vi "InstrumentSelection.vi"(8 "error in (no error)":errorcluster, 9 "Verify GPIB address":bool, 10 "Instrument type":T1(ring), 11 "Instrument name IN":string(combo)) -> (0 "error out":errorcluster, 1 "Instrument name OUT":string, 2 "LCR":refnum<class "LCRControl.lvclass">, 3 "Supply":refnum<class "SupplyControl.lvclass">, 4 "Switching":refnum<class "Switching.lvclass">, 5 "Multimeter":refnum<class "MultimeterControl.lvclass">)   [LabVIEW 2019, in "InstrControl.lvclass"]
uses:
  InstrControl.lvclass
  SupplyControl/SupplyControl.lvclass
  C:/Users/Semiprobe/Desktop/Probe-Test-Software/itk-strip-sensor-qc/LabVIEW 2019/InstrControl/InstrControl.lvclass
  LCRControl/LCRControl.lvclass
  MultimeterControl/MultimeterControl.lvclass
  Switching/Switching.lvclass
  SupplyControl/Keithley 2410/KE2410.lvclass
  C:/Users/Semiprobe/Desktop/Probe-Test-Software/itk-strip-sensor-qc/LabVIEW 2019/InstrControl/SupplyControl/SupplyControl.lvclass
  SupplyControl/Keithley 2657A/KE2657A.lvclass
  SupplyControl/Keithley 6517/KE6517.lvclass
  SupplyControl/Keithley 487/KE487.lvclass
  SupplyControl/Keithley 236 & 237/KE236.lvclass
  LCRControl/WK6440B/WK6440B.lvclass
  C:/Users/Semiprobe/Desktop/Probe-Test-Software/itk-strip-sensor-qc/LabVIEW 2019/InstrControl/LCRControl/LCRControl.lvclass
  LCRControl/WK6425/WK6425.lvclass
  MultimeterControl/Keithley 2000/KE2000.lvclass
  C:/Users/Semiprobe/Desktop/Probe-Test-Software/itk-strip-sensor-qc/LabVIEW 2019/InstrControl/MultimeterControl/MultimeterControl.lvclass
  Switching/Pickering/Pickering.lvclass
  C:/Users/Semiprobe/Desktop/Probe-Test-Software/itk-strip-sensor-qc/LabVIEW 2019/InstrControl/Switching/Switching.lvclass
  Switching/Keithley 3706A/KE3706A.lvclass
  Switching/LXIPXISwitching/LXIPXISwitching.lvclass
  InstrumentSetup.vi
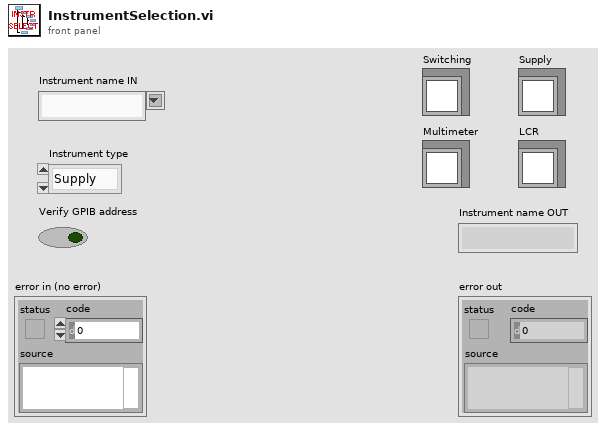
[diagram p1: front panel]
types:
  T1 = enum16{"Supply", "LCR", "Multimeter", "Switching"}
  T2 = cluster{"KE 2410":cluster{"Instrument name":string, "address":refnum<visa-resource-name>, "Instrument type":u16}, "KE 6517":cluster{"Instrument name":string, "address":refnum<visa-resource-name>, "Instrument type":u16}, "KE 487":cluster{"Instrument name":string, "address":refnum<visa-resource-name>, "Instrument type":u16}, "KE 236":cluster{"Instrument name":string, "address":refnum<visa-resource-name>, "Instrument type":u16}, "WK 6440B":cluster{"Instrument name":string, "address":refnum<visa-resource-name>, "Instrument type":u16}, "WK 6425":cluster{"Instrument name":string, "address":refnum<visa-resource-name>, "Instrument type":u16}, "Pickering Matrix":cluster{"Instrument name":string, "address":refnum<visa-resource-name>, "Instrument type":u16}, "KE 2000":cluster{"Instrument name":string, "address":refnum<visa-resource-name>, "Instrument type":u16}, "KE3706A Switching":cluster{"Instrument name":string, "address":refnum<visa-resource-name>, "Instrument type":u16}, "KE 2657A":cluster{"Instrument name":string, "address":refnum<visa-resource-name>, "Instrument type":u16}}
  T3 = cluster{"Current Limit":sgl, "KE2410":refnum<class "KE2410.lvclass">}
  T4 = cluster{"Current Limit":sgl, "KE2657A":refnum<class "KE2657A.lvclass">}
  T5 = cluster{"Current Limit":u16, "KE6517":refnum<class "KE6517.lvclass">}
  T6 = cluster{"Compliance":u16, "Range:":u16, "KE487":refnum<class "KE487.lvclass">}
  T7 = cluster{"current \ncompliance level":dbl, "compliance/\nmeasurement range (auto:0)":u16, "KE236":refnum<class "KE236.lvclass">}
  T8 = cluster{"RC Configuration":u16, "AC amplitude [V]":dbl, "AC frequency [Hz]":i32, "WK6440B":refnum<class "WK6440B.lvclass">}
  T9 = cluster{"RC Configuration":u16, "AC amplitude [V]":dbl, "AC frequency [Hz]":i32, "WK6425":refnum<class "WK6425.lvclass">}
  T10 = cluster{"Range":u16, "Range Value":dbl, "Function":u16, "KE2000":refnum<class "KE2000.lvclass">}
  T11 = cluster{"Matrix address":string, "Mux1 address":string, "Mux2 address":string, "Pickering":refnum<class "Pickering.lvclass">, "Matrix X Channels":cluster{"Bias Supply / SMU LO":i32, "Bias Supply / SMU HI":i32, "CV Box LO":i32, "CV Box HI":i32, "CV Box LO IN":i32, "CV Box HI IN":i32, "Volt meter LO":i32, "Volt meter HI":i32, "Mux1 C1":i32, "Mux1 C2":i32, "Mux2 C1":i32, "Mux2 C2":i32}}
  T12 = cluster{"Mux1 slot":string, "Mux2 slot":string, "KE3706A":refnum<class "KE3706A.lvclass">}
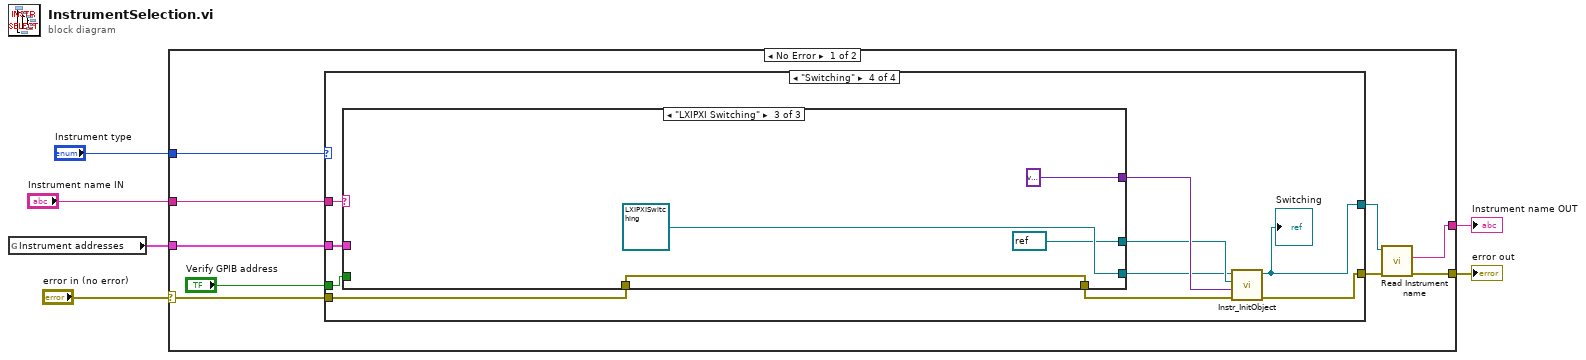
[diagram p0: block diagram]
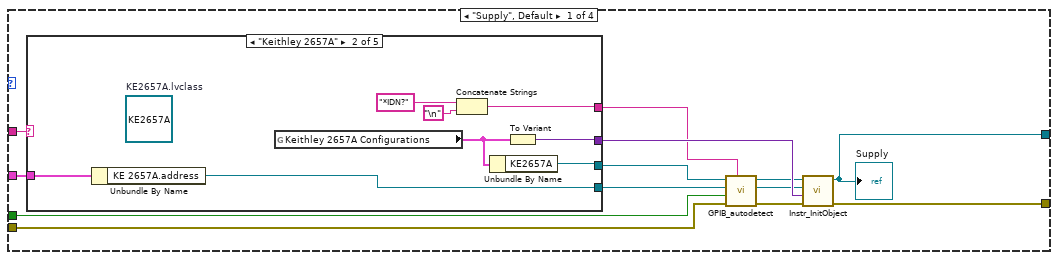
[diagram p2: hidden frame]
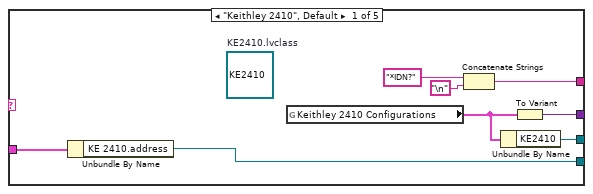
[diagram p3: hidden frame]
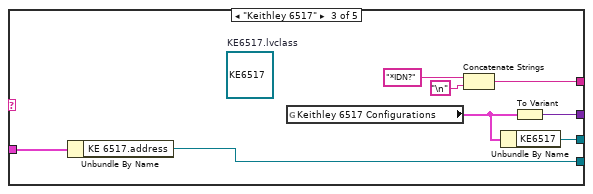
[diagram p4: hidden frame]
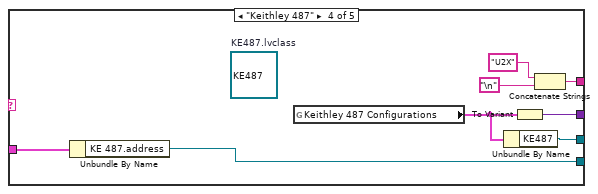
[diagram p5: hidden frame]
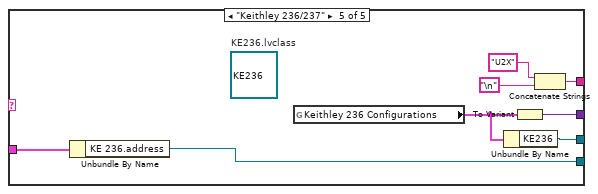
[diagram p6: hidden frame]
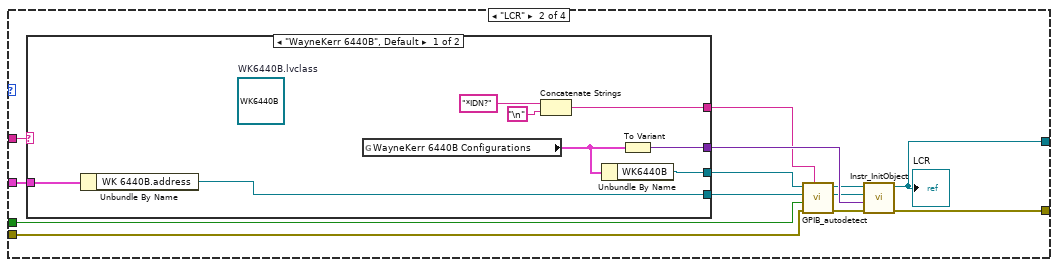
[diagram p7: hidden frame]
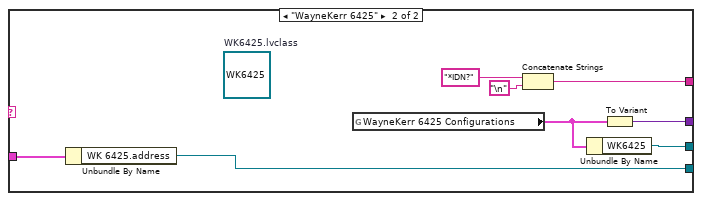
[diagram p8: hidden frame]
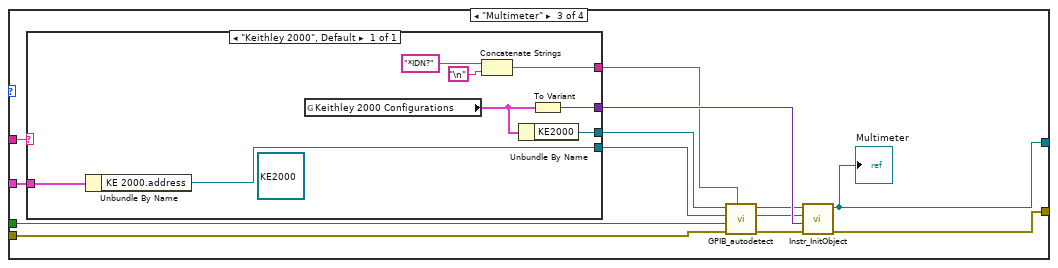
[diagram p9: hidden frame]
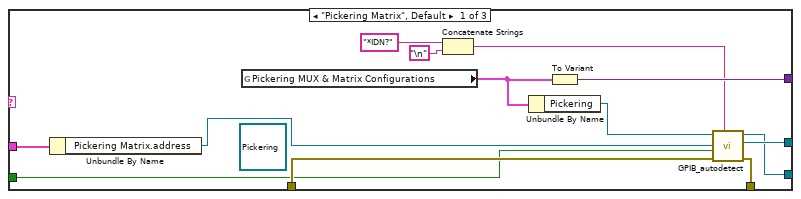
[diagram p10: hidden frame]
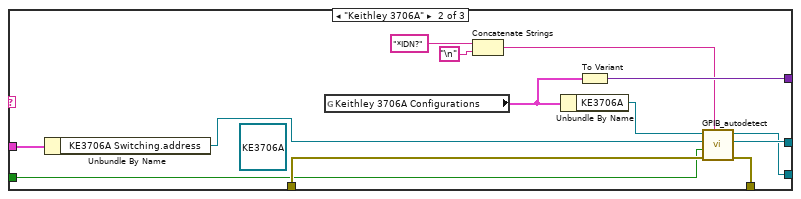
[diagram p11: hidden frame]
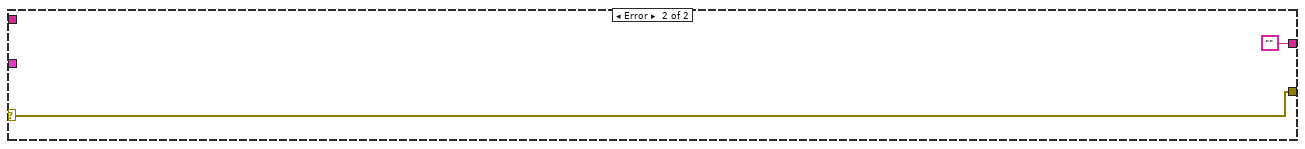
[diagram p12: hidden frame]
diagram:
  n1 = global read "InstrumentSetup.vi" "Instrument addresses"() -> (w1:T2)
  n2 = case shown="No Error" "error in (no error)" {
    selector: "error in (no error)" -> [w13 w160]
    tunnel: [w14 w160] -> w5
    tunnel: [w15 ""] -> w4
    tunnel: "Instrument type" -> [w10 _]
    tunnel: "Instrument name IN" -> [w9 _]
    tunnel: w1 -> [w8 _]
    frame No Error {
      n3 = case shown="\"Switching\"" w10 {
        tunnel: w9 -> [w28 w81 w110 w125]
        tunnel: [w27 w79 w108 w127] -> w12
        tunnel: w13 -> [w19 w76 w100 w123]
        tunnel: [w26 w80 w109 w128] -> w11
        tunnel: w8 -> [w25 w78 w107 w126]
        tunnel: "Verify GPIB address" -> [w18 w70 w105 w122]
        frame "Supply", Default {
          n4 = case shown="\"Keithley 2657A\"" w28 {
            tunnel: [w33 w39 w48 w56 w64] -> w21
            tunnel: w25 -> [w36 w38 w52 w60 w68]
            tunnel: [w35 w37 w51 w59 w67] -> w23
            tunnel: [w34 w40 w50 w58 w66] -> w24
            tunnel: [w29 w41 w45 w53 w61] -> w16
            frame "Keithley 2410", Default {
              (unwired) refnum<class "KE2410.lvclass"> refnum  # KE2410.lvclass
              n5 = Unbundle By Name(w36) -> ("KE 2410.address"=w35:refnum<visa-resource-name>)
              n6 = global read "InstrumentSetup.vi" "Keithley 2410 Configurations"() -> (w32:T3)
              n7 = Concatenate Strings("*IDN?" ("regular expression"), "\n") -> (w29:string)
              n8 = Unbundle By Name(w32) -> ("KE2410"=w33:refnum<class "KE2410.lvclass">)
              n9 = To Variant(anything=w32) -> (Variant=w34:variant)
            }
            frame "Keithley 2657A" {
              (unwired) refnum<class "KE2657A.lvclass"> refnum  # KE2657A.lvclass
              n10 = Unbundle By Name(w38) -> ("KE 2657A.address"=w37:refnum<visa-resource-name>)
              n11 = global read "InstrumentSetup.vi" "Keithley 2657A Configurations"() -> (w44:T4)
              n12 = Concatenate Strings("*IDN?" ("regular expression"), "\n") -> (w41:string)
              n13 = Unbundle By Name(w44) -> ("KE2657A"=w39:refnum<class "KE2657A.lvclass">)
              n14 = To Variant(anything=w44) -> (Variant=w40:variant)
            }
            frame "Keithley 6517" {
              (unwired) refnum<class "KE6517.lvclass"> refnum  # KE6517.lvclass
              n15 = Unbundle By Name(w52) -> ("KE 6517.address"=w51:refnum<visa-resource-name>)
              n16 = global read "InstrumentSetup.vi" "Keithley 6517 Configurations"() -> (w49:T5)
              n17 = Concatenate Strings("*IDN?" ("regular expression"), "\n") -> (w45:string)
              n18 = Unbundle By Name(w49) -> ("KE6517"=w48:refnum<class "KE6517.lvclass">)
              n19 = To Variant(anything=w49) -> (Variant=w50:variant)
            }
            frame "Keithley 487" {
              (unwired) refnum<class "KE487.lvclass"> refnum  # KE487.lvclass
              n20 = Unbundle By Name(w60) -> ("KE 487.address"=w59:refnum<visa-resource-name>)
              n21 = global read "InstrumentSetup.vi" "Keithley 487 Configurations"() -> (w57:T6)
              n22 = Unbundle By Name(w57) -> ("KE487"=w56:refnum<class "KE487.lvclass">)
              n23 = To Variant(anything=w57) -> (Variant=w58:variant)
              n24 = Concatenate Strings("U2X" ("regular expression"), "\n") -> (w53:string)
            }
            frame "Keithley 236/237" {
              (unwired) refnum<class "KE236.lvclass"> refnum  # KE236.lvclass
              n25 = Unbundle By Name(w68) -> ("KE 236.address"=w67:refnum<visa-resource-name>)
              n26 = global read "InstrumentSetup.vi" "Keithley 236 Configurations"() -> (w65:T7)
              n27 = Unbundle By Name(w65) -> ("KE236"=w64:refnum<class "KE236.lvclass">)
              n28 = To Variant(anything=w65) -> (Variant=w66:variant)
              n29 = Concatenate Strings("U2X" ("regular expression"), "\n") -> (w61:string)
            }
          }
          n30 = call-dynamic "GPIB_autodetect.vi"("ID command"=w16, "error in (no error)"=w19, "Verify GPIB address"=w18, "Instrument address in"=w23, "InstrControl in"=w21) -> ("error out"=w17:errorcluster, "Instrument address out"=w22:refnum<visa-resource-name>, "InstrControl out"=w20:refnum<class "SupplyControl.lvclass">)  [unwired: 4 in]
          n31 = call-dynamic "Instr_InitObject.vi"("error in (no error)"=w17, "Instrument Configuration"=w24, "Instrument address"=w22, "SupplyControl in"=w20) -> ("error out"=w26:errorcluster, "SupplyControl out"=w27:refnum<class "SupplyControl.lvclass">)  [unwired: 6 in]
          "Supply" <- w27
        }
        frame "LCR" {
          n32 = case shown="\"WayneKerr 6440B\", Default" w81 {
            tunnel: [w85 w93] -> w72
            tunnel: w78 -> [w89 w97]
            tunnel: [w88 w96] -> w74
            tunnel: [w87 w95] -> w77
            tunnel: [w82 w90] -> w69
            frame "WayneKerr 6440B", Default {
              (unwired) refnum<class "WK6440B.lvclass"> refnum  # WK6440B.lvclass
              n33 = Unbundle By Name(w89) -> ("WK 6440B.address"=w88:refnum<visa-resource-name>)
              n34 = global read "InstrumentSetup.vi" "WayneKerr 6440B Configurations"() -> (w86:T8)
              n35 = Concatenate Strings("*IDN?" ("regular expression"), "\n") -> (w82:string)
              n36 = Unbundle By Name(w86) -> ("WK6440B"=w85:refnum<class "WK6440B.lvclass">)
              n37 = To Variant(anything=w86) -> (Variant=w87:variant)
            }
            frame "WayneKerr 6425" {
              (unwired) refnum<class "WK6425.lvclass"> refnum  # WK6425.lvclass
              n38 = Unbundle By Name(w97) -> ("WK 6425.address"=w96:refnum<visa-resource-name>)
              n39 = global read "InstrumentSetup.vi" "WayneKerr 6425 Configurations"() -> (w94:T9)
              n40 = Concatenate Strings("*IDN?" ("regular expression"), "\n") -> (w90:string)
              n41 = Unbundle By Name(w94) -> ("WK6425"=w93:refnum<class "WK6425.lvclass">)
              n42 = To Variant(anything=w94) -> (Variant=w95:variant)
            }
          }
          n43 = call-dynamic "GPIB_autodetect.vi"("ID command"=w69, "error in (no error)"=w76, "Verify GPIB address"=w70, "Instrument address in"=w74, "InstrControl in"=w72) -> ("error out"=w75:errorcluster, "Instrument address out"=w73:refnum<visa-resource-name>, "InstrControl out"=w71:refnum<class "LCRControl.lvclass">)  [unwired: 4 in]
          n44 = call-dynamic "Instr_InitObject.vi"("error in (no error)"=w75, "Instrument Configuration"=w77, "Instrument address"=w73, "LCRControl in"=w71) -> ("error out"=w80:errorcluster, "LCRControl out"=w79:refnum<class "LCRControl.lvclass">)  [unwired: 6 in]
          "LCR" <- w79
        }
        frame "Multimeter" {
          n45 = case shown="\"Keithley 2000\", Default" w110 {
            tunnel: [w114] -> w101
            tunnel: w107 -> [w118]
            tunnel: [w117] -> w104
            tunnel: [w116] -> w106
            tunnel: [w111] -> w98
            frame "Keithley 2000", Default {
              (unwired) refnum<class "KE2000.lvclass"> refnum ("KE2000.lvclass")
              n46 = Unbundle By Name(w118) -> ("KE 2000.address"=w117:refnum<visa-resource-name>)
              n47 = global read "InstrumentSetup.vi" "Keithley 2000 Configurations"() -> (w115:T10)
              n48 = Concatenate Strings("*IDN?" ("regular expression"), "\n") -> (w111:string)
              n49 = Unbundle By Name(w115) -> ("KE2000"=w114:refnum<class "KE2000.lvclass">)
              n50 = To Variant(anything=w115) -> (Variant=w116:variant)
            }
          }
          n51 = call-dynamic "GPIB_autodetect.vi"("ID command"=w98, "error in (no error)"=w100, "Verify GPIB address"=w105, "Instrument address in"=w104, "InstrControl in"=w101) -> ("error out"=w99:errorcluster, "Instrument address out"=w103:refnum<visa-resource-name>, "InstrControl out"=w102:refnum<class "KE2000.lvclass">)  [unwired: 4 in]
          n52 = call-dynamic "Instr_InitObject.vi"("error in (no error)"=w99, "Instrument Configuration"=w106, "Instrument address"=w103, "KE2000 in"=w102) -> ("error out"=w109:errorcluster, "KE2000 out"=w108:refnum<class "KE2000.lvclass">)  [unwired: 6 in]
          "Multimeter" <- w108
        }
        frame "Switching" {
          n53 = case shown="\"LXIPXI Switching\"" w125 {
            tunnel: w126 -> [w141 w152 _]
            tunnel: [w139 w151 variant ("Variant")] -> w124
            tunnel: w123 -> [w135 w149 w155]
            tunnel: w122 -> [w134 w142 _]
            tunnel: [w131 w148 w155] -> w121
            tunnel: [w130 w145 refnum<visa-resource-name> refnum ("Instrument address out")] -> w120
            tunnel: [w129 w144 refnum<class "LXIPXISwitching.lvclass"> refnum ("LXIPXISwitching.lvclass")] -> w119
            frame "Pickering Matrix", Default {
              (unwired) refnum<class "Pickering.lvclass"> refnum ("Pickering")
              n54 = Unbundle By Name(w141) -> ("Pickering Matrix.address"=w133:refnum<visa-resource-name>)
              n55 = global read "InstrumentSetup.vi" "Pickering MUX & Matrix Configurations"() -> (w140:T11)
              n56 = Concatenate Strings("*IDN?" ("regular expression"), "\n") -> (w136:string)
              n57 = Unbundle By Name(w140) -> ("Pickering"=w132:refnum<class "Pickering.lvclass">)
              n58 = To Variant(anything=w140) -> (Variant=w139:variant)
              n59 = call-dynamic "GPIB_autodetect.vi"("ID command"=w136, "error in (no error)"=w135, "Verify GPIB address"=w134, "Instrument address in"=w133, "InstrControl in"=w132) -> ("error out"=w131:errorcluster, "Instrument address out"=w130:refnum<visa-resource-name>, "InstrControl out"=w129:refnum<class "Pickering.lvclass">)  [unwired: 4 in]
            }
            frame "Keithley 3706A" {
              (unwired) refnum<class "KE3706A.lvclass"> refnum ("KE3700A in")
              n60 = Unbundle By Name(w152) -> ("KE3706A Switching.address"=w146:refnum<visa-resource-name>)
              n61 = global read "InstrumentSetup.vi" "Keithley 3706A Configurations"() -> (w154:T12)
              n62 = Concatenate Strings("*IDN?" ("regular expression"), "\n") -> (w143:string)
              n63 = Unbundle By Name(w154) -> ("KE3706A"=w147:refnum<class "KE3706A.lvclass">)
              n64 = To Variant(anything=w154) -> (Variant=w151:variant)
              n65 = call-dynamic "GPIB_autodetect.vi"("ID command"=w143, "error in (no error)"=w149, "Verify GPIB address"=w142, "Instrument address in"=w146, "InstrControl in"=w147) -> ("error out"=w148:errorcluster, "Instrument address out"=w145:refnum<visa-resource-name>, "InstrControl out"=w144:refnum<class "KE3706A.lvclass">)  [unwired: 4 in]
            }
            frame "LXIPXI Switching" {
            }
          }
          n66 = call-dynamic "Instr_InitObject.vi"("error in (no error)"=w121, "Instrument Configuration"=w124, "Instrument address"=w120, "Switching in"=w119) -> ("error out"=w128:errorcluster, "Switching out"=w127:refnum<class "Switching.lvclass">)  [unwired: 6 in]
          "Switching" <- w127
        }
      }
      n67 = call-dynamic "Read Instrument name.vi"("error in (no error)"=w11, "InstControl in"=w12) -> ("error out"=w14:errorcluster, "Instrument name"=w15:string)  [unwired: 7 in, 1 out]
    }
    frame Error {
    }
  }
  "error out" <- w5
  "Instrument name OUT" <- w4
